vi "Examples Washer Testing.vi"() -> ()   [LabVIEW 2009]
uses:
  GEA2 Washer Interface Ctrl.ctl
panel:
  in  "Tab Control":enum32{"Example 1: Version"}(tab)
  out "WriteOK":bool
  out "Number of Responses":i32
  out "Version Found":bool
  out "Version Information":u8[](array[numeric])
  # "[0]-   Major_Version_Firmware\n[1]-   Minor_Version_Firmware\n[2]-   Major_Version_CriticalCode\n[3]-   Minor_Version_CriticalCode\n[4]-   Major_Version_ParametricData\n[5]-   Minor_Version_ParametricData\n[6]-   Major_Version_Inverter\n[7]-   Minor_Version_Inverter\n[8]-   Major_Version_InverterCritical\n[9]-   Minor_Version_InverterCritical\n[10]-   Major_Version_MachineControl\n[11]-   Minor_Version_MachineControl\n[12]-   Major_Version_MachineControlCritical\n[13]-   Minor_Version_MachineControlCritical\n[14]-   Major_Version_MachineControlEeprom\n[15]-   Minor_Version_MachineControlEeprom"
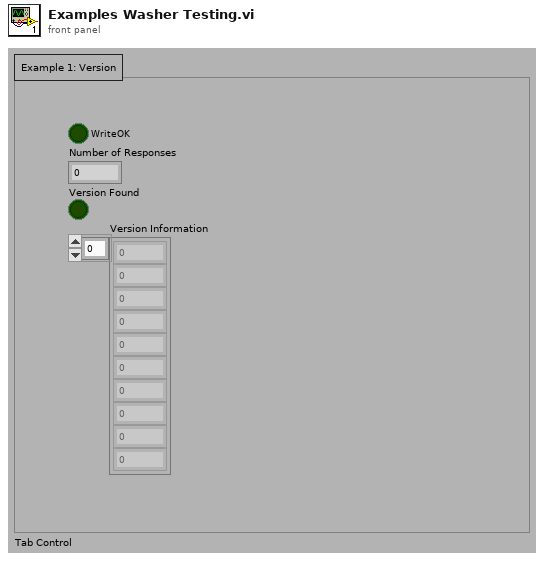
[diagram p1: front panel]
types:
  T1 = typedef "GEA2 Washer Interface Ctrl.ctl" = enum16{"Init Com Port", "SendCMD", "ReadPort", "Close Port", "Send Byte Data", "Read Continuous"}
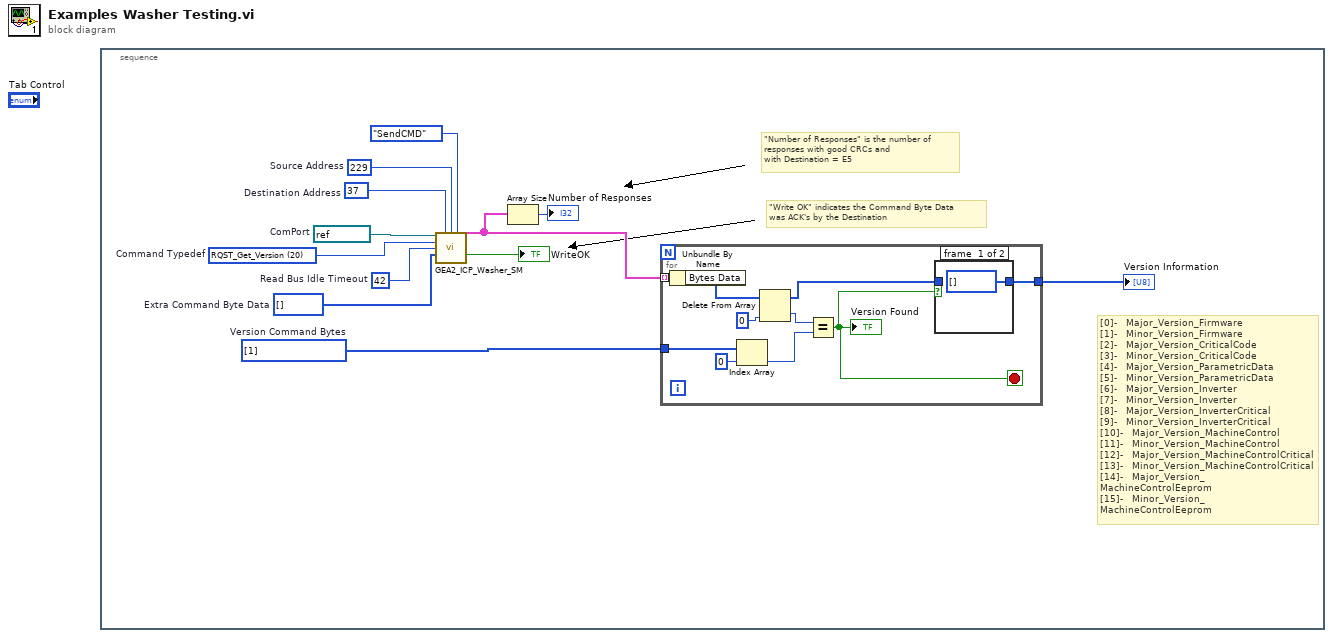
[diagram p0: block diagram]
diagram:
  n1 = stacked-sequence {
    frame #0 {
      w1 = u32 42  # Read Bus Idle Timeout
      w2 = u8[] []  # Extra Command Byte Data
      w3 = u8 20 items=["CMD_Entry_Command", "CMD_Load_Control", "RQST_Input_Status", "CMD_LED_Control", "RQST_Encoder_Position_Status", "RQST_A2D_Status", "RQST_Switch_States_Status", "CMD_Buzzer_Control", "CMD_Shift_to_Spin", "CMD_Shift_to_Agitate", "RQST_Mode_Shift_Complete_Status", "CMD_Control_Inverter", "CMD_Spin_Action", "CMD_Agitate_Action", "RQST_Total_Switch_Status", "RQST_Total_Encoder_Status", "CMD_Test_Eeprom", "RQST_Eeprom_Test_Status", "CMD_Power_Mode", "RQST_Error_Status", "RQST_Get_Version", "CMD_Set_Personality", "RQST_Get_Personality", "CMD_Serial_Number", "RQST_Serial_Number_Status", "CMD_Model_Number", "RQST_Model_Number_Status", "CMD_Enter_Boot_Loader"]  # Command Typedef
      w6 = u8[] [1]  # Version Command Bytes
      w10 = refnum<visa-resource-name> "COM1"  # ComPort
      w11 = u8 229  # Source Address
      w12 = u8 37  # Destination Address
      # "[0]-   Major_Version_Firmware\n[1]-   Minor_Version_Firmware\n[2]-   Major_Version_CriticalCode\n[3]-   Minor_Version_CriticalCode\n[4]-   Major_Version_ParametricData\n[5]-   Minor_Version_ParametricData\n[6]-   Major_Version_Inverter\n[7]-   Minor_Version_Inverter\n[8]-   Major_Version_InverterCritical\n[9]-   Minor_Version_InverterCritical\n[10]-   Major_Version_MachineControl\n[11]-   Minor_Version_MachineControl\n[12]-   Major_Version_MachineControlCritical\n[13]-   Minor_Version_MachineControlCritical\n[14]-   Major_Version_MachineControlEeprom\n[15]-   Minor_Version_MachineControlEeprom"
      # "\"Write OK\" indicates the Command Byte Data\nwas ACK's by the Destination"
      # "\"Number of Responses\" is the number of\nresponses with good CRCs and\nwith Destination = E5"
      n2 = call "GEA2_ICP_Washer_SM.vi"("ComPort"=w10, "Destination Address"=w12, "Source Address"=w11, "Mode"=GEA2_Washer_Interface_Ctrl."SendCMD", "Command"=w3, "Read Bus Idle Timeout"=w1, "Byte Data"=w2) -> ("Good Responses"=w7:cluster{"Bytes Data":u8[]}[], "WriteOK"=→"WriteOK":bool)  [unwired: 5 in, 2 out]
      n3 = Array Size(array=w7) -> (size(s)=→"Number of Responses":i32)
      n4 = for {
        tunnel: w7 -> [w22] mode=indexing
        tunnel: w6 -> [w18]
        tunnel: [w15] -> w5
        stop <- w16 stop-if-true
        n5 = Unbundle By Name(w22) -> ("Bytes Data"=w14:u8[])
        n6 = Index Array(array=w18, index=0) -> (element=w17:u8)
        n7 = Delete From Array(array=w14, index=0) -> (deleted portion=w20:u8, array with subset deleted=w13:u8[])  [unwired: 1 in]
        n8 = Equal?(x=w20, y=w17) -> (x = y?=w16:bool)
        "Version Found" <- w16
        n9 = case shown="True" w16 {
          tunnel: [u8[] [] ("Bytes Data") w24] -> w15
          tunnel: w13 -> [_ w24]
          frame #0 {
          }
          frame #1 {
          }
        }
      }
      "Version Information" <- w5
    }
  }
